vi "tircomcomd.vi"() -> ()   [LabVIEW 2020]
uses:
  <vilib>/MakerHub/LINX/Public/Peripherals/Digital/Digital Write N Chans.vi
  <vilib>/MakerHub/LINX/Public/Peripherals/Analog/Analog Read 1 Chan.vi
  <vilib>/MakerHub/LINX/Private/Local IO/LinxDigitalWrite.vi
  <vilib>/MakerHub/LINX/Public/Utilities/Check Channel.vi
  <vilib>/MakerHub/LINX/Public/Peripherals/Analog/Analog Read N Chans.vi
  <vilib>/MakerHub/LINX/Private/Local IO/LinxAnalogRead.vi
  <vilib>/MakerHub/LINX/Public/Utilities/Open Serial.vi
  <vilib>/MakerHub/LINX/Private/Utilties/Generate Error.vi
  <vilib>/MakerHub/LINX/LMH-LINX.lvlib
panel:
  out "Voltage":dbl
  out "Error Out":errorcluster
  in  "Serial Port":refnum<visa-resource-name>="COM51"
  in  "stop":bool
  in  "Values":bool[](array[boolean])=[FALSE, FALSE, FALSE, FALSE, FALSE, FALSE, FALSE, FALSE, FALSE]
  out "Numeric":i32
  # "relais blanc\nSN23-41-08"
  # "relais noir\nSN23-41-08"
  # "R4 3P4S\n\n______________\n\nR5 3P4S Led\n\nR6 2P6S Led\n\nR3 3P4S\n\nR2 2P6S\n\n_\n\n_\n\nR1 2P6S\n\n_\n\n_\n\n_\n\n\n_"
  # "R1 CAN3P46\n\nR2 CAN2P6S\n\nR3 CAN2P6S\n\nR4 CAN3P4S\n\nR5 LED3P4S\n\nR6 LED2P6S"
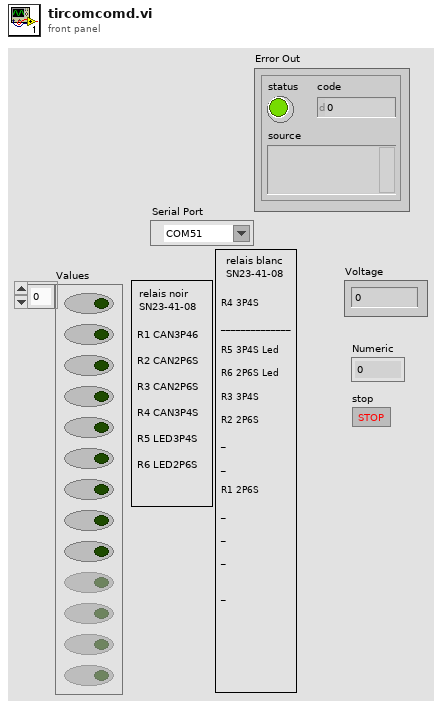
[diagram p1: front panel]
types:
  T1 = typedef "LMH-LINX.lvlib/LINX Ref.ctl" = cluster{"IO":T2, "Interface":T3, "LINX Device Config":T4}
  T2 = typedef "LMH-LINX.lvlib/Platform.ctl" = enum16{"Remote", "Local"}
  T3 = typedef "LMH-LINX.lvlib/Interface.ctl" = enum16{"Serial", "TCP"}
  T4 = typedef "LMH-LINX.lvlib/Device.lvlib/LINX Device Config.ctl" = cluster{"Interface":T3, "COM Port":refnum<visa-resource-name>, "TCP Configuration":T5, "Device Family":u8, "Device ID":u8, "Device Name":string, "TCP Ref":refnum<k5>, "Channels":T6}
  T5 = typedef "LMH-LINX.lvlib/Device.lvlib/TCP Config.ctl" = cluster{"IP Address":string, "Port":u16}
  T6 = typedef "LMH-LINX.lvlib/Channels.ctl" = cluster{"DI":u8[], "DO":u8[], "AI":u8[], "AO":u8[], "PWM":u8[], "QE":u8[], "UART":u8[], "I2C 2":u8[], "SPI":u8[], "CAN":u8[], "Servo":u8[], "AI Ref (V)":dbl, "AI Resolution (Bits)":u8, "AO Ref (V)":dbl, "AO Resolution (Bits)":u8}
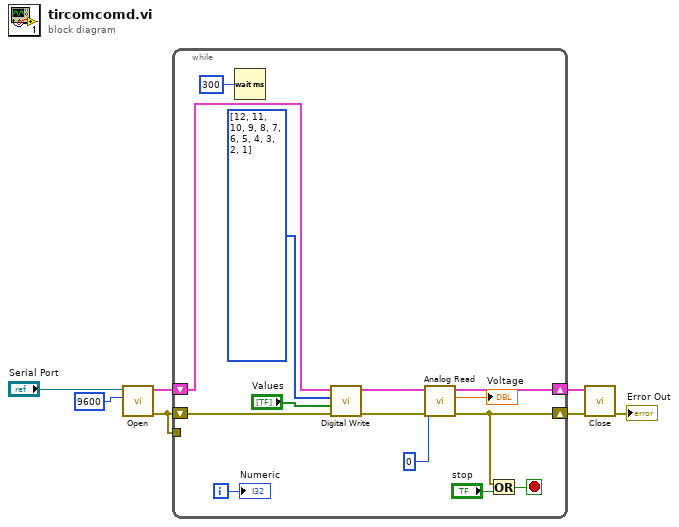
[diagram p0: block diagram]
diagram:
  n1 = call-poly <vilib>:"Open.vi"("Baud Rate Override"=u32 9600, "Serial Port"="Serial Port") -> ("Error Out"=w1:errorcluster, "LINX Resource"=w4:T1)  [unwired: 7 in, 1 out]
  n2 = while {
    shift-right: [w10] -> w5
    shift-left: w1 -> [w21]
    shift-right: [w12] -> w3
    shift-left: w4 -> [w20]
    tunnel: w1 -> [_]
    i -> [w18]
    stop <- w14 stop-if-true
    n3 = Wait (ms)(milliseconds to wait=u32 300) -> ()  [unwired: 1 out]
    n4 = call-poly <vilib>:"Digital Write.vi"("Error In"=w21, "Values"="Values", "DO Channels"=u8[] [12, 11, 10, 9, 8, 7, 6, 5, 4, 3, 2, 1], "LINX Resource"=w20) -> ("Error Out"=w11:errorcluster, "LINX Resource"=w13:T1)  [unwired: 6 in]
    n5 = call-poly <vilib>:"Analog Read.vi"("Error In"=w11, "Analog Channel"=u8 0, "LINX Resource"=w13) -> ("Error Out"=w10:errorcluster, "Voltage"=→"Voltage":dbl, "LINX Resource"=w12:T1)  [unwired: 5 in, 1 out]
    n6 = Or(x=w10, y="stop") -> (x .or. y?=w14:bool)
    "Numeric" <- w18
  }
  n7 = call <vilib>:"Close.vi"("Error In"=w5, "LINX Resource"=w3) -> ("Error Out"=→"Error Out":errorcluster)  [unwired: 9 in]
